vi "AddControl.vi"(8 "error in (no error)":errorcluster, 9 "CtlRef":refnum<vi>, 10 "CtlName":string, 11 "CtlLookup In":T1) -> (0 "error out":errorcluster, 3 "CtlLookup Out":T1)   [LabVIEW 2020, in "CtlReferences.lvlib" / "CtlReferences.lvclass"]
doc: "Add control specified by cluster to CtlLookup"
uses:
  CtlReferences.lvclass
  TypeDefs/CtlLookup.ctl
  CtlReferences.lvclass/CtlReferences.ctl
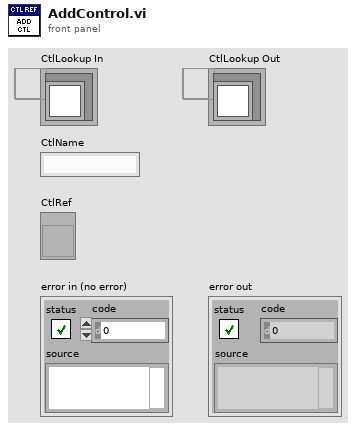
[diagram p1: front panel]
types:
  T1 = typedef "CtlReferences.lvlib/CtlReferences.lvclass/CtlLookup.ctl" = refnum<data-value>
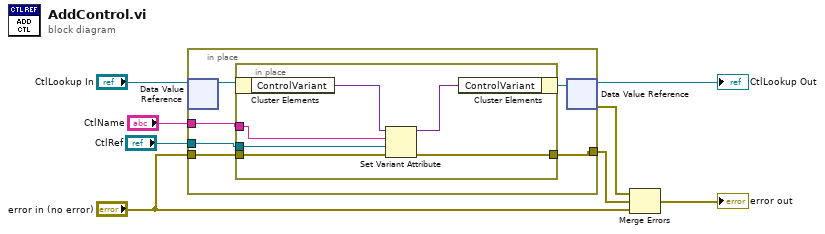
[diagram p0: block diagram]
diagram:
  n1 = in-place {
    in-place-border: "CtlRef" -> [w11]
    in-place-border: [w9] -> w5
    in-place-border: "CtlName" -> [w12]
    in-place-border: "error in (no error)" -> [w10]
    n2 = in-place-dvr #1("CtlLookup In") -> (w14:refnum<class "CtlReferences.lvclass">)  [unwired: 1 out]
    n3 = in-place {
      in-place-border: w11 -> [w17]
      in-place-border: [w18] -> w9
      in-place-border: w10 -> [w16]
      in-place-border: w12 -> [w15]
      n4 = in-place-cluster #2(w14) -> ("ControlVariant"=w20:variant)
      n5 = Set Variant Attribute(Variant=w20, name=w15, value=w17, error in=w16) -> (Variant out=w19:variant, error out=w18:errorcluster)  [unwired: 1 out]
      n6 = in-place-cluster #2("ControlVariant"=w19) -> (w13:refnum<class "CtlReferences.lvclass">)
    }
    n7 = in-place-dvr #1(w13) -> (→"CtlLookup Out":T1, w4:errorcluster)
  }
  n8 = Merge Errors(w4, w5, "error in (no error)") -> (→"error out":errorcluster)
